vi "UHR-Fleezers Control (fpga) - 9.1.vi"() -> ()   [LabVIEW 2009]
doc: "UHR-Fleezers Instrument Control Code (fpga)"
uses:
  <vilib>/Platform/TimedLoop/XDataNode/XDataNode.xnode
  <vilib>/Platform/TimedLoop/XDataNode/loadlvalarms.vi
  <vilib>/Platform/TimedLoop/XDataNode/timing_clust.ctl
  <vilib>/Platform/TimedLoop/XDataNode/nitl_modes.ctl
  <vilib>/Platform/TimedLoop/XDataNode/wakeup.ctl
  <vilib>/eio/EIOMethodNode/EIOMethodNode.xnode
  <vilib>/rvi/eio/nirviEIOMethodImplementation/nirviEIOMethodImplementation.xnode
  <vilib>/rvi/eio/common/nirviEmuTemplateMethod_noerrors.vi
  <vilib>/rvi/eio/common/nirviEmuClasses.ctl
  <vilib>/eio/EIONode/EIONode.xnode
  <vilib>/rvi/eio/nirviEIOImplementation/nirviEIOImplementation.xnode
  <vilib>/rvi/DataTransferAndStorage/Container/XNode/niFpgaContainer.xnode
  <vilib>/rvi/interface/RandomDataEmulation/niFpgaRandomDataHandleErrors.vi
  <vilib>/rvi/interface/RandomDataEmulation/nirviRandomDataFPGAFIFO.vi
  <vilib>/rvi/DataTransferAndStorage/Container/Common/niFpgaContainerMethod.ctl
  <vilib>/rvi/DataTransferAndStorage/Container/Common/niFpgaTransferTypeControl.ctl
  <vilib>/Platform/TimedLoop/XDataNode/XDNodeRunTimeDep.lvlib
panel:
  in  "Tab Control":T1(tab)=enum."Green Laser Interlacing"
  in  "AI Averages":u16=1 min=1 step=1
  in  "AI1 Sets to FIFO":T2={"Set 1"=TRUE, "Set 2"=TRUE, "Set 3"=FALSE}
  in  "N of AI1 Int Acq Sets":i16=2 min=1 max=3 step=1
  out "Number of AI channels":i16
  out "AI Late Counter":u32
  in  "ai count":u32=400
  out "AI late?":bool
  in  "+ phase":bool
  in  "Phase count adjustment":i16
  out "Relative phase":i16
  in  "DMA buffer timeout":i32
  in  "AI to FIFO":bool
  in  "Tab Control 2":T3(tab)
  in  "Swap F1 and F2":bool
  in  "Freq or Amp switch first":bool=TRUE
  in  "Cont. Scan":bool
  in  "Abort scan":bool
  in  "Cycles per step":u64
  in  "Scan BD":bool
  in  "Number of scans":u16
  in  "Scan steps":u64
  in  "Scan freq.  increment":i64
  out "Scanning":bool
  in  "Start scan":bool
  in  "OSK Bd 1":bool
  in  "Reset Bd 1":bool
  in  "RD":bool
  in  "PMODE":bool
  in  "OSK Bd 2":bool
  in  "Reset Bd 2":bool
  in  "Direct RF Box \nCommunication":bool
  in  "Data BD 2":u8 format="%08b"
  in  "Data BD 1":u8 format="%08b"
  in  "Address":u8 format="%02x"
  in  "Update Data":bool
  in  "FPGA Controls\n RF Box":bool
  in  "Number Interlace Cycles":u8=2 min=1 max=3
  in  "Interlace Off Parameters":u8=1 min=1 max=3
  in  "Interlace ON/OFF":bool
  out "DIO Relative phase":i16
  in  "Phase count adjustment (DIO)":i16
  in  "+ phase (DIO)":bool
  out "DIO Late Counter":u32
  out "DIO Late?":bool
  in  "DIO count 1 (ticks)":u32=400
  in  "DIO count 2 (ticks)":u32=400
  in  "DIO count 3 (ticks)":u32=400
  out "AI2 Y Sum Set 2":i16
  out "AI2 Y Sum Set 1":i16
  in  "FB Gains Set 1":T4={"proportional gain (Kc)"=10, "integral gain (Kc*Ts/Ti)"=5, "derivative gain (Kc*Td/Ts)"=0}
  in  "FB Setpoint Set 1":i16 min=0 step=1
  in  "FB Reset Set 1":bool
  in  "FB On/Off Set 1":bool
  in  "FB Reset Set 2":bool
  in  "FB On/Off Set 2":bool
  in  "FB Setpoint Set 2":i16 min=0 step=1
  in  "FB Gains Set 2":T4={"proportional gain (Kc)"=10, "integral gain (Kc*Ts/Ti)"=5, "derivative gain (Kc*Td/Ts)"=0}
  in  "FB output range 2":cluster{"output high":i16, "output low":i16}={"output high"=3000, "output low"=0}
  in  "FB output range 1":cluster{"output high":i16, "output low":i16}={"output high"=3000, "output low"=0}
  out "Scan I":u64
  in  "Amp switch delay":u16=5
  in  "Freq switch delay":u16
  in  "BD 2 Amplitude 1":u16
  in  "BD 1 Amplitude 1":u16
  in  "BD 2 Frequency 1":u64
  in  "BD 1 Frequency 1":u64
  in  "BD 2 Amplitude 2":u16
  in  "BD 1 Amplitude 2":u16
  in  "BD 2 Frequency 2":u64
  in  "BD 1 Frequency 2":u64
  in  "BD 2 Amplitude 3":u16
  in  "BD 1 Amplitude 3":u16
  in  "BD 2 Frequency 3":u64
  in  "BD 1 Frequency 3":u64
  out "Numeric":i32
  out "AO2 2":i16
  out "AO1 2":i16
  in  "1D or 2D Scan?":bool
  in  "Abort scan (MCL)":bool
  in  "MCL Scan Axis":bool
  in  "Cont. Scan (MCL)":bool
  out "Scan I (MCL)":u64
  in  "Number of scans (MCL)":u16
  out "Scanning MCL":bool
  in  "Scan steps (MCL)":u64
  in  "Cycles per step (MCL)":u64
  in  "Scan freq.  increment (MCL)":i16
  in  "Start scan (MCL)":bool
  in  "AO2":i16
  in  "AO1":i16
  out "MCL Late Counter":u32
  out "MCL Late?":bool
  in  "MCL count":u32=800
  out "MCL Relative Phase":i16
  in  "Phase count adjustment (MCL)":i16
  in  "+ phase (MCL)":bool
  in  "APD Gate Operating Mode":u8 max=2 step=1
  in  "Invert APD Gate":bool
  in  "APD Gate OFF Count":u32=100
  in  "APD Gate ON Count":u32=300
  out "APD Gate Late Counter":u32
  out "APD Gate Late?":bool
  out "APD Gate Relative Phase":i16
  in  "Phase count adjustment (APD Gate)":i16
  in  "+ phase (APD Gate)":bool
  out "APD 2 Counts 0":u32
  out "APD 2 Counts 1":u32
  out "APD 1 Counts 0":u32
  out "APD 1 Counts 1":u32
  out "APD out state":bool
  in  "APD 2 AO offset":i16
  in  "APD 1 AO offset":i16
  in  "APD 2 AO scale factor":i16=1
  in  "APD 1 AO scale factor":i16=1
  in  "APD to FIFO":bool
  in  "APD Acq Rate Count":u32=20000000
  out "APD Acq Late Counter":u32
  out "APD Acq Late?":bool
  out "APD Acq Relative Phase":i16
  in  "Phase Count Adjustment (APD Acq)":i16
  in  "+ phase (APD Acq)":bool
  out "Green FB Signals":T5
  in  "Green FB Count":u32=1200
  out "Green Late Counter":u32
  out "Green FB Late?":bool
  out "Green FB Relative Phase":i16
  in  "Phase count adjustment (Green FB)":i16=10
  in  "+ phase (Green FB)":bool
  out "Green FB Sum":i16
  in  "Green int current ON count adj":u32=150
  in  "Current Out":u16=30000
  in  "Green FB On/Off":bool
  in  "Green FB Setpoint":i16=250 min=0 step=1
  in  "Green FB Gains":T4={"proportional gain (Kc)"=10, "integral gain (Kc*Ts/Ti)"=5, "derivative gain (Kc*Td/Ts)"=0}
  in  "Green FB Reset":bool
  in  "Operating Mode 2":u8=2 max=2 step=1
  in  "Invert GI 2":bool
  in  "Green interlace OFF count 2":u32=900
  in  "Green interlace ON count 2":u32=300
  out "GI Late Counter 2":u32
  out "GI Late? 2":bool
  out "GI Relative phase 2":i16
  in  "Phase count adjustment (GI) 2":i16=20
  in  "+ phase (GI) 2":bool
  in  "Green interlace OFF count":u32=100
  out "GI Relative phase":i16
  in  "Phase count adjustment (GI)":i16
  in  "+ phase (GI)":bool
  out "GI Late?":bool
  in  "Green interlace ON count":u32=300
  out "GI Late Counter":u32
  in  "Invert GI":bool
  in  "Operating Mode":u8 max=2 step=1
  # "Only one of these can be on\nat a time:"
  # "Raster Scan AOD"
  # "1 (X)"
  # "2 (Y)"
  # "IR Intensity Feedback (RF BD 1)"
  # "AO1 (Y)"
  # "2D"
  # "1D"
  # "AO2 (X)"
  # "APD AO for aligning"
  # "Detection Loop"
  # "Green fluorescent laser digital gate interlacing loop"
  # "0 Forced ON\n1 Forced OFF\n2 Interlacing"
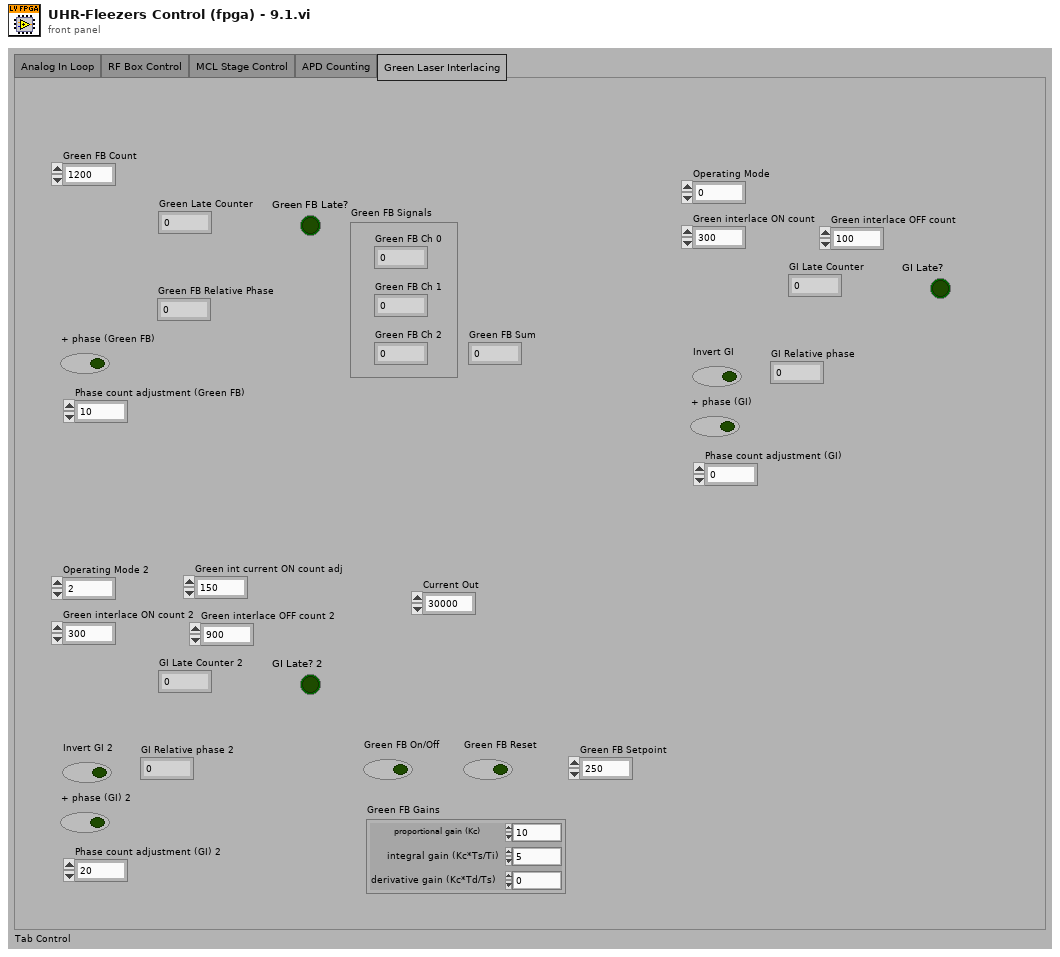
[diagram p1: front panel]
types:
  T1 = enum32{"Analog In Loop", "RF Box Control", "MCL Stage Control", "APD Counting", "Green Laser Interlacing"}
  T2 = cluster{"Set 1":bool, "Set 2":bool, "Set 3":bool}
  T3 = enum32{"Controls", "Interlacing Frequency and Amplitude Values"}
  T4 = cluster{"proportional gain (Kc)":i16, "integral gain (Kc*Ts/Ti)":i16, "derivative gain (Kc*Td/Ts)":i16}
  T5 = cluster{"Green FB Ch 0":i16, "Green FB Ch 1":i16, "Green FB Ch 2":i16}
  T6 = typedef "nirviEmuClasses.ctl" = enum16{"IO Read", "IO Write", "Method", "Property Read", "Property Write"}
  T7 = typedef "XDNodeRunTimeDep.lvlib/timing_clust.ctl" = cluster{"Expected End [f-1]":u64, "Actual End [f-1]":u64, "Finished Late? [f-1]":bool, "Expected End [i-1]":u64, "Actual End [i-1]":u64, "Finished Late? [i-1]":bool, "Expected Start [i]":u64, "Actual Start [i]":u64, "Expected Start [f]":u64, "Actual Start [f]":u64, "Source Name":string, "Structure Name":string, "Period":i64, "Deadline":i64, "Offset":i64, "Start":i64, "Priority":i32, "Timeout":i32, "Mode":T8, "Wakeup Reason":T9, "Error":errorcluster, "Source Type":string, "Secondary Source Type":string, "Global End Time":u64, "Global Start Time":u64, "Frame Duration":u64, "Iteration Duration":u64, "Assigned CPU":i32, "I/O Scan Engine Mode":u32}
  T8 = typedef "XDNodeRunTimeDep.lvlib/nitl_modes.ctl" = enum32{"No Change", "Process missed periods, maintain original phase", "Discard missed periods, maintain original phase", "Process missed periods, ignore original phase", "Discard missed periods, ignore original phase"}
  T9 = typedef "XDNodeRunTimeDep.lvlib/wakeup.ctl" = enum32{"Normal", "Aborted", "Asynchronous wakeup", "Timing source error", "Timed loop error", "Timeout"}
  T10 = typedef "niFpgaContainerMethod.ctl" = enum16{"Write", "Read", "Clear", "Get Number of Elements to Write", "Get Number of Elements to Read", "Enable", "Disable", "Flush and Disable", "Get Stream State"}
  T11 = typedef "niFpgaTransferTypeControl.ctl" = enum16{"Target-Scoped", "Host to Target - DMA", "Target to Host - DMA", "Peer to Peer Reader", "Peer to Peer Writer", "Bidirectional"}
  T12 = cluster{"Chassis2/Mod1/AI0":i16, "Chassis2/Mod1/AI1":i16, "Chassis2/Mod1/AI2":i16}
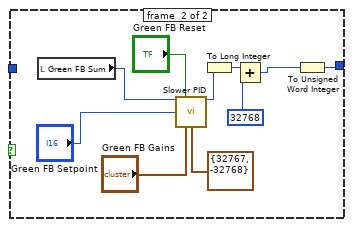
[diagram p2: hidden frame]
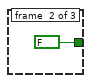
[diagram p3: hidden frame]
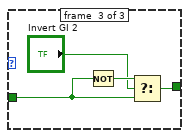
[diagram p4: hidden frame]
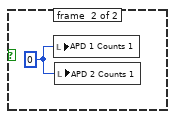
[diagram p5: hidden frame]
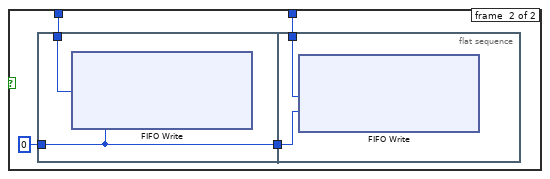
[diagram p6: hidden frame]
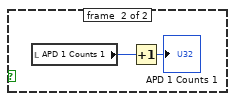
[diagram p7: hidden frame]
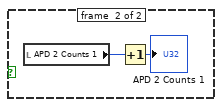
[diagram p8: hidden frame]
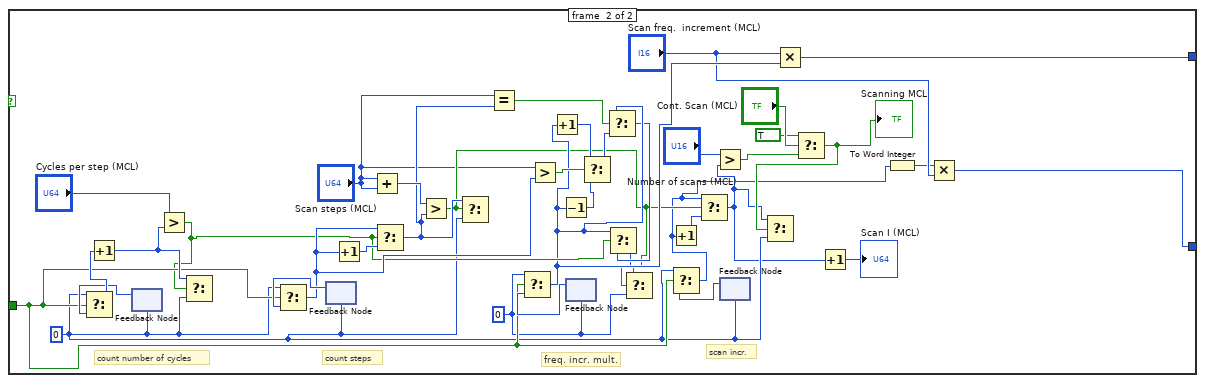
[diagram p9: hidden frame]
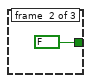
[diagram p10: hidden frame]
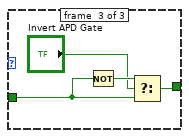
[diagram p11: hidden frame]
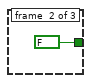
[diagram p12: hidden frame]
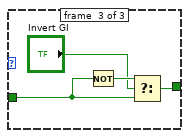
[diagram p13: hidden frame]
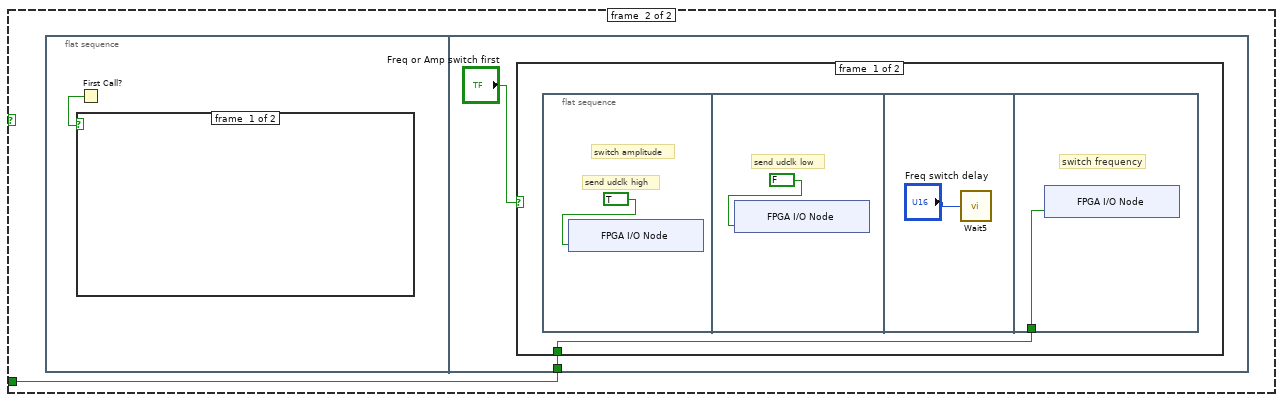
[diagram p14: hidden frame]
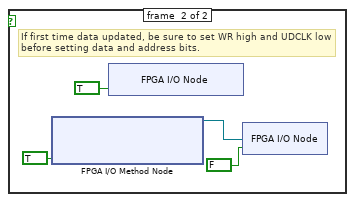
[diagram p15: hidden frame]
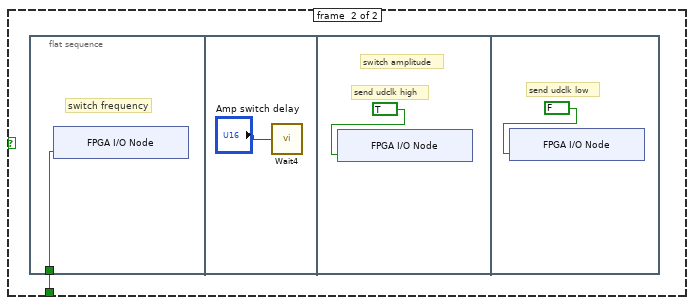
[diagram p16: hidden frame]
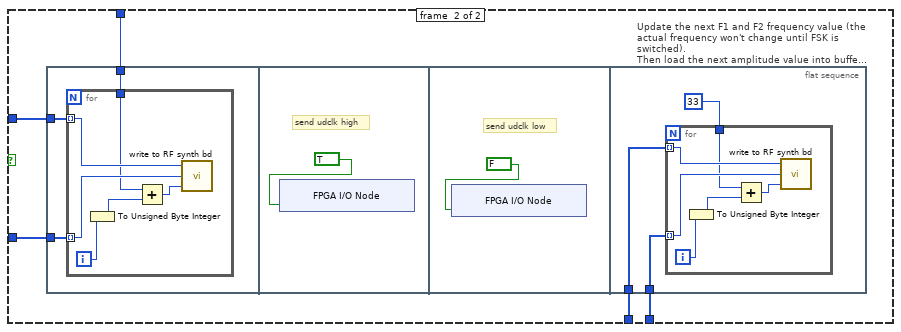
[diagram p17: hidden frame]
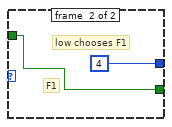
[diagram p18: hidden frame]
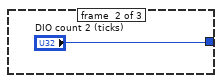
[diagram p19: hidden frame]
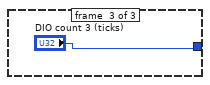
[diagram p20: hidden frame]
diagram:
  # "timing array current index"
  # "timing array"
  # "timing counter (phase adjusted here)"
  # "late counter"
  n1 = flat-sequence "FPGA initialization to do before running any of the loops" {
    tunnel: [u32 0 ("DIO count 3 (ticks)")] -> w1
    tunnel: [w10] -> _
    frame #0 {
      # "This is a kludge to let host programs know how many channels of data are in the DMA stream.  Set by hand."
      # "Start up expansion chassis early\nto avoid delays later"
      # "This pin controls udclk on the RF boards.\nWhen initially configuring the boards, this pin needs to be\nconfigured as a high impedance input.  Later it will be switched\nto an output."
      # "Initial setting of DIO data and \naddress to low (before reset).  \nThis needs to happen before the other\ncontrol method loops execute."
      n2 = xnode "FPGA I/O Node"("Chassis2/Mod4/AO0"=u16 0) -> ("Chassis2/Mod1/AI0"=w10:i16)  [unwired: 2 in, 2 out]
      n3 = xnode "FPGA I/O Method Node"("Enable"=FALSE) -> ()  [unwired: 1 in, 1 out]
      n4 = xnode "FPGA I/O Node"("Connector1/DIO0"=FALSE, "Connector1/DIO1"=FALSE, "Connector1/DIO2"=FALSE, "Connector1/DIO3"=FALSE, "Connector1/DIO4"=FALSE, "Connector1/DIO5"=FALSE, "Connector1/DIO6"=FALSE, "Connector1/DIO7"=FALSE, "Connector1/DIO8"=FALSE, "Connector1/DIO9"=FALSE, "Connector1/DIO10"=FALSE, "Connector1/DIO11"=FALSE, "Connector1/DIO12"=FALSE, "Connector1/DIO13"=FALSE, "Connector1/DIO15"=FALSE, "Connector1/DIO20"=FALSE, "Connector1/DIO21"=FALSE, "Connector1/DIO22"=FALSE, "Connector1/DIO23"=FALSE, "Connector1/DIO24"=FALSE, "Connector1/DIO25"=FALSE, "Connector1/DIO26"=FALSE, "Connector1/DIO27"=FALSE, "Connector1/DIO14"=FALSE) -> ()  [unwired: 24 in, 24 out]
      "Number of AI channels" <- i16 12 ("Number of AI channels")
    }
  }
  n5 = node-c288() -> (w3:T7)  [unwired: 1 in]
  n6 = local read "AO1"() -> (w5:i16)
  n7 = local read "AO2"() -> (w4:i16)
  n8 = timed-loop "RF box board DIO control: control bits" {
    timing: w3 -> [_]
    timing-out: [_] -> w2
    tunnel: [w393] -> _
    tunnel: w1 -> [w393]
    stop <- FALSE stop-if-true
    n9 = xnode "FPGA I/O Node"("Connector1/DIO16"="RD", "Connector1/DIO17"="PMODE", "Connector1/DIO18"="OSK Bd 1", "Connector1/DIO19"="Reset Bd 1", "Connector1/DIO28"="OSK Bd 2", "Connector1/DIO29"="Reset Bd 2") -> ()  [unwired: 6 in, 6 out]
  }
  n10 = while "DAQ AI set 1" {
    shift-right: [w481] -> _
    shift-left: w1 -> [w486]
    stop <- FALSE stop-if-true
    n11 = flat-sequence {
      tunnel: w486 -> [w496]
      tunnel: [w497] -> w484
      tunnel: [w496] -> w483
      tunnel: [w507] -> w494
      tunnel: [w506] -> w493
      tunnel: [w505] -> w492
      tunnel: [w504] -> w491
      tunnel: [w503] -> w490
      tunnel: [w502] -> w489
      tunnel: [w501] -> w488
      tunnel: [w500] -> w487
      tunnel: [w499] -> w485
      tunnel: w484 -> [w499]
      tunnel: w483 -> [w498]
      tunnel: [w498] -> w482
      tunnel: [w684] -> w481
      tunnel: w494 -> [w722]
      tunnel: w493 -> [w721]
      tunnel: w492 -> [w705]
      tunnel: w491 -> [w720]
      tunnel: w490 -> [w709]
      tunnel: w489 -> [w708]
      tunnel: w488 -> [w707]
      tunnel: w487 -> [w706]
      tunnel: w485 -> [w701]
      tunnel: w482 -> [w698]
      frame #0 {
        n12 = call "Loop Timer3"("Count(Ticks)"=w496) -> ("Tick Count(Ticks)"=w497:u32)
      }
      frame #1 {
        n13 = xnode "FPGA I/O Node"("Connector1/DIO31"=TRUE ("Connector1/DIO33")) -> ("Connector0/AI0"=w507:i16, "Connector0/AI1"=w506:i16, "Connector0/AI2"=w505:i16, "Connector0/AI3"=w504:i16, "Connector0/AI4"=w503:i16, "Connector0/AI5"=w502:i16, "Connector0/AI6"=w501:i16, "Connector0/AI7"=w500:i16)  [unwired: 9 in, 9 out]
      }
      frame #2 {
        # "Adjust phase after data acquired if button pressed"
        n14 = feedback #1(i16 1) -> (w713:i16)
        n15 = Increment(x=w713) -> (x+1=w719:i16)
        n16 = Greater?(x=w719, y="N of AI1 Int Acq Sets") -> (0:w716:bool)
        n17 = Select(t=i16 1, s=w716, f=w719) -> (s? t:f=w718:i16)
        n18 = feedback #2(FALSE ("AI to FIFO")) -> (w703:bool)
        n19 = case shown="1, Default" w713 {
          tunnel: w705 -> [w725 w729 _]
          tunnel: "AI1 Sets to FIFO" -> [w727 w731 w734]
          tunnel: [w726 w730 w733] -> w710
          tunnel: ["AI to FIFO" w728 w732] -> w702
          tunnel: w703 -> [_ w728 w732]
          frame #0 {
            n20 = Unbundle By Name(w727) -> ("Set 1"=w726:bool)
            "AI2 Y Sum Set 1" <- w725
          }
          frame #1 {
            n21 = Unbundle By Name(w731) -> ("Set 2"=w730:bool)
            "AI2 Y Sum Set 2" <- w729
          }
          frame #2 {
            n22 = Unbundle By Name(w734) -> ("Set 3"=w733:bool)
          }
        }
        n23 = And(x=w710, y=w702) -> (x .and. y?=w712:bool)
        n24 = case shown="True" w712 {
          tunnel: w722 -> [_ w739]
          tunnel: w721 -> [_ w740]
          tunnel: w705 -> [_ w741]
          tunnel: w720 -> [_ w742]
          tunnel: w709 -> [_ w746]
          tunnel: w708 -> [_ w745]
          tunnel: w707 -> [_ w744]
          tunnel: w706 -> [_ w743]
          frame #0 {
          }
          frame #1 {
            n25 = Greater?(x="AI Averages", y=u16 1) -> (0:w737:bool)
            n26 = case shown="True" w737 {
              tunnel: w746 -> [w757 w814]
              tunnel: w745 -> [w756 w813]
              tunnel: w744 -> [w755 w812]
              tunnel: w743 -> [w754 w811]
              tunnel: w742 -> [w753 w810]
              tunnel: w741 -> [w758 w809]
              tunnel: w740 -> [w759 w808]
              tunnel: w739 -> [w760 w807]
              tunnel: "AI Averages" -> [_ w794]
              tunnel: "DMA buffer timeout" -> [w748 w791]
              frame #0 {
                n27 = Join Numbers(hi=w760, lo=w759) -> ((hi.lo)=w752:u32)
                n28 = Join Numbers(hi=w758, lo=w753) -> ((hi.lo)=w751:u32)
                n29 = Join Numbers(hi=w757, lo=w756) -> ((hi.lo)=w750:u32)
                n30 = Join Numbers(hi=w755, lo=w754) -> ((hi.lo)=w749:u32)
                n31 = Build Array(w752, w751, w750, w749) -> (w747:u32[])
                n32 = for {
                  tunnel: w747 -> [w762] mode=indexing
                  tunnel: w748 -> [w763]
                  n33 = To Unsigned Long Integer(number=w762) -> (unsigned 32bit integer=w761:u32)
                  n34 = xnode ("FIFO Write")("Element"=w761, "Timeout"=w763) -> ()  [unwired: 1 in, 2 out]
                }
              }
              frame #1 {
                w798 = u16 0
                n35 = To Long Integer(number=w807) -> (32bit integer=w800:i32)
                n36 = To Long Integer(number=w808) -> (32bit integer=w817:i32)
                n37 = To Long Integer(number=w809) -> (32bit integer=w816:i32)
                n38 = To Long Integer(number=w810) -> (32bit integer=w815:i32)
                n39 = To Long Integer(number=w814) -> (32bit integer=w806:i32)
                n40 = To Long Integer(number=w813) -> (32bit integer=w805:i32)
                n41 = To Long Integer(number=w812) -> (32bit integer=w804:i32)
                n42 = To Long Integer(number=w811) -> (32bit integer=w803:i32)
                n43 = Build Array(w800, w817, w816, w815, w806, w805, w804, w803) -> (w789:i32[])
                n44 = feedback #3(w789) -> (w802:i32[])
                n45 = Add(x=w789, y=w802) -> (x+y=w801:i32[])
                n46 = feedback #4(w798) -> (w796:u16)
                n47 = Increment(x=w796) -> (x+1=w793:u16)
                n48 = Equal?(x=w793, y=u16 1) -> (x = y?=w792:bool)
                n49 = Select(t=w789, s=w792, f=w801) -> (s? t:f=w790:i32[])
                n50 = Greater Or Equal?(x=w793, y=w794) -> (x >= y?=w795:bool)
                n51 = Select(t=w798, s=w795, f=w793) -> (s? t:f=w797:u16)
                n52 = case shown="True" w795 {
                  tunnel: w790 -> [_ w819]
                  tunnel: w791 -> [_ w818]
                  frame #0 {
                  }
                  frame #1 {
                    n53 = for {
                      tunnel: w819 -> [w821] mode=indexing
                      tunnel: w818 -> [w822]
                      n54 = To Unsigned Long Integer(number=w821) -> (unsigned 32bit integer=w820:u32)
                      n55 = xnode ("FIFO Write")("Element"=w820, "Timeout"=w822) -> ()  [unwired: 1 in, 2 out]
                    }
                  }
                }
              }
            }
          }
        }
        n56 = feedback #5(w701) -> (w700:u32)
        n57 = Subtract(x=w701, y=w700) -> (x-y=w699:u32)
        n58 = Subtract(x=w699, y=w698) -> (x-y=w695:u32)
        n59 = Subtract(x="ai count", y=w695) -> (x-y=w685:u32)
        n60 = Greater?(x=w695, y=u32 0) -> (0:w693:bool)
        "AI late?" <- w693
        n61 = feedback #6(u32 0) -> (w691:u32)
        n62 = Increment(x=w691) -> (x+1=w690:u32)
        n63 = Select(t=w690, s=w693, f=w691) -> (s? t:f=w692:u32)
        "AI Late Counter" <- w692
        n64 = xnode "I/O Node"("Connector1/DIO31"=FALSE ("Connector1/DIO34")) -> ()  [unwired: 1 in, 1 out]
        n65 = Boolean To (0,1)(Boolean="+ phase") -> (0, 1=w687:i16)
        n66 = Multiply(x=w687, y="Phase count adjustment") -> (x*y=w681:i16)
        n67 = feedback #7(i16 0) -> (w683:i16)
        n68 = Add(x=w685, y=w681) -> (x+y=w684:u32)
        n69 = Subtract(x=w683, y=w681) -> (x-y=w682:i16)
        "Relative phase" <- w682
      }
    }
  }
  n70 = while "APD 1 Counter" {
    tunnel: w1 -> [_]
    stop <- FALSE stop-if-true
    n71 = flat-sequence {
      frame #0 {
        n72 = xnode "FPGA I/O Method Node"("FPGA I/O In"=refnum<k21> "Connector0/DIO10" ("APD 1 DO"), "Timeout"=-1) -> ()  [unwired: 2 out]
      }
      frame #1 {
        n73 = local read "APD out state"() -> (w887:bool)
        n74 = case shown="False" w887 {
          frame #0 {
            n75 = local read "APD 1 Counts 0"() -> (w889:u32)
            n76 = Increment(x=w889) -> (x+1=→"APD 1 Counts 0":u32)
          }
          frame #1 {
            n77 = local read "APD 1 Counts 1"() -> (w891:u32)
            n78 = Increment(x=w891) -> (x+1=→"APD 1 Counts 1":u32)
          }
        }
      }
    }
  }
  n79 = while "APD 2 Counter" {
    tunnel: w1 -> [_]
    stop <- FALSE stop-if-true
    n80 = flat-sequence {
      frame #0 {
        n81 = xnode "FPGA I/O Method Node"("FPGA I/O In"=refnum<k21> "Connector0/DIO11" ("APD 2 DO"), "Timeout"=-1) -> ()  [unwired: 2 out]
      }
      frame #1 {
        n82 = local read "APD out state"() -> (w918:bool)
        n83 = case shown="False" w918 {
          frame #0 {
            n84 = local read "APD 2 Counts 0"() -> (w920:u32)
            n85 = Increment(x=w920) -> (x+1=→"APD 2 Counts 0":u32)
          }
          frame #1 {
            n86 = local read "APD 2 Counts 1"() -> (w922:u32)
            n87 = Increment(x=w922) -> (x+1=→"APD 2 Counts 1":u32)
          }
        }
      }
    }
  }
  n88 = while "RF box board DIO control: parallel communication" {
    shift-right: [w929] -> _
    shift-left: w1 -> [w928]
    shift-right: [w927] -> _
    shift-left: FALSE ("Swap F1 and F2") -> [w926]
    stop <- FALSE stop-if-true
    n89 = flat-sequence {
      tunnel: w926 -> [w933]
      tunnel: w928 -> [w931]
      tunnel: [w933] -> w925
      tunnel: [w932] -> w924
      tunnel: [w931] -> w923
      tunnel: [w939] -> w929
      tunnel: [w938] -> w927
      tunnel: w925 -> [w937]
      tunnel: w924 -> [w935]
      tunnel: w923 -> [w934]
      frame #0 {
        n90 = call "Loop Timer"("Count(Ticks)"=w931) -> ("Tick Count(Ticks)"=w932:u32)
      }
      frame #1 {
        n91 = flat-sequence {
          tunnel: ["FPGA Controls\n RF Box"] -> w936
          tunnel: w937 -> [w940]
          tunnel: [w1089] -> w939
          tunnel: [w1109] -> w938
          tunnel: w936 -> [w1108]
          tunnel: w935 -> [w1102]
          tunnel: w934 -> [w1099]
          frame #0 {
            n92 = case shown="True" "FPGA Controls\n RF Box" {
              tunnel: w940 -> [_ w942]
              frame #0 {
              }
              frame #1 {
                n93 = flat-sequence {
                  tunnel: w942 -> [w987]
                  frame #0 {
                    n94 = First Call?() -> (First Call?: T/F=w943:bool)
                    n95 = case shown="True" w943 {
                      frame #0 {
                      }
                      frame #1 {
                        # "If first time data updated, be sure to set WR high and UDCLK low\nbefore setting data and address bits."
                        n96 = xnode "FPGA I/O Method Node"("Enable"=TRUE) -> ("FPGA I/O Out"=w945:refnum<k21>)  [unwired: 1 in]
                        n97 = xnode "FPGA I/O Node"("Connector1/DIO15"=TRUE) -> ()  [unwired: 1 in, 1 out]
                        n98 = xnode "FPGA I/O Node"("I/O Item"=FALSE ("Connector1/DIO30"), "FPGA I/O In"=w945) -> ()  [unwired: 1 out]
                      }
                    }
                  }
                  frame #1 {
                    n99 = case shown="True" "Freq or Amp switch first" {
                      tunnel: w987 -> [w989 w1033]
                      frame #0 {
                        n100 = flat-sequence {
                          tunnel: w989 -> [w1019]
                          frame #0 {
                            # "switch amplitude"
                            # "send udclk high"
                            n101 = xnode "FPGA I/O Node"("Connector1/DIO30"=TRUE ("Connector1/DIO15")) -> ()  [unwired: 1 in, 1 out]
                          }
                          frame #1 {
                            # "send udclk low"
                            n102 = xnode "FPGA I/O Node"("Connector1/DIO30"=FALSE ("Connector1/DIO15")) -> ()  [unwired: 1 in, 1 out]
                          }
                          frame #2 {
                            n103 = call "Wait5"("Count(Ticks)"="Freq switch delay") -> ()  [unwired: 1 out]
                          }
                          frame #3 {
                            # "switch frequency"
                            n104 = xnode "FPGA I/O Node"("Connector1/DIO36"=w1019) -> ()  [unwired: 1 in, 1 out]
                          }
                        }
                      }
                      frame #1 {
                        n105 = flat-sequence {
                          tunnel: w1033 -> [w1034]
                          frame #0 {
                            # "switch frequency"
                            n106 = xnode "FPGA I/O Node"("Connector1/DIO36"=w1034) -> ()  [unwired: 1 in, 1 out]
                          }
                          frame #1 {
                            n107 = call "Wait4"("Count(Ticks)"="Amp switch delay") -> ()  [unwired: 1 out]
                          }
                          frame #2 {
                            # "switch amplitude"
                            # "send udclk high"
                            n108 = xnode "FPGA I/O Node"("Connector1/DIO30"=TRUE ("Connector1/DIO15")) -> ()  [unwired: 1 in, 1 out]
                          }
                          frame #3 {
                            # "send udclk low"
                            n109 = xnode "FPGA I/O Node"("Connector1/DIO30"=FALSE ("Connector1/DIO15")) -> ()  [unwired: 1 in, 1 out]
                          }
                        }
                      }
                    }
                  }
                }
              }
            }
          }
          frame #1 {
            # "This is the prior cycle's on time"
            # "increment timing\nindex, reset to 0 if \nend of matrix"
            # "Reset to begginning (1) when number of cycles reached."
            # "timing index"
            # "build byte stacks for writing data\n(must correspond to addresses array constant)"
            # "Timing housekeeping"
            # "Adjust phase if late\n(maintains constant phase relationship between cycles)"
            n110 = feedback #8(u8 0 ("t")) -> (w1105:u8)
            n111 = Increment(x=w1105) -> (x+1=w1149:u8)
            n112 = Increment(x="Number Interlace Cycles") -> (x+1=w1144:u8)
            n113 = Equal?(x=w1149, y=w1144) -> (x = y?=w1151:bool)
            n114 = Select(t=u8 1, s=w1151, f=w1149) -> (s? t:f=w1104:u8)
            n115 = Increment(x=w1104) -> (x+1=w1146:u8)
            n116 = Equal?(x=w1146, y=w1144) -> (x = y?=w1147:bool)
            n117 = Select(t=u8 1, s=w1147, f=w1146) -> (s? t:f=w1143:u8)
            n118 = Select(t=w1143, s="Interlace ON/OFF", f="Interlace Off Parameters") -> (s? t:f=w1127:u8)
            n119 = case shown="1, Default" w1127 {
              tunnel: [w1223 "BD 1 Frequency 2" "BD 1 Frequency 3"] -> w1139
              tunnel: [w1222 "BD 2 Frequency 2" "BD 2 Frequency 3"] -> w1128
              tunnel: ["BD 2 Amplitude 1" "BD 2 Amplitude 2" "BD 2 Amplitude 3"] -> w1077
              tunnel: [w1211 w1281 "BD 1 Amplitude 3"] -> w1080
              frame #0 {
                w1218 = u8 0 ("f")
                n120 = local read "Scanning"() -> (w1224:bool)
                n121 = Or(x=w1224, y="Start scan") -> (x .or. y?=w1216:bool)
                n122 = Not(x="Abort scan") -> (.not. x?=w1214:bool)
                n123 = And(x=w1214, y=w1216) -> (x .and. y?=w1213:bool)
                n124 = case "Raster scan" shown="True" w1213 {
                  tunnel: [i16 0 w1270] -> w1219
                  tunnel: "Start scan" -> [_ w1255]
                  frame #0 {
                    n125 = local write "Scanning"(FALSE ("scanning")) -> ()
                  }
                  frame #1 {
                    w1239 = i64 0
                    w1238 = u64 0
                    # "scan incr."
                    # "freq. incr. mult."
                    # "count steps"
                    # "count number of cycles"
                    n126 = feedback #9(w1238) -> (w1267:u64)
                    n127 = Select(t=w1238, s=w1255, f=w1267) -> (s? t:f=w1269:u64)
                    n128 = Increment(x=w1269) -> (x+1=w1266:u64)
                    n129 = Greater?(x="Cycles per step", y=w1266) -> (0:w1248:bool)
                    n130 = Select(t=w1266, s=w1248, f=w1238) -> (s? t:f=w1265:u64)
                    n131 = feedback #10(w1238) -> (w1264:u64)
                    n132 = Select(t=w1238, s=w1255, f=w1264) -> (s? t:f=w1259:u64)
                    n133 = Increment(x=w1259) -> (x+1=w1263:u64)
                    n134 = Add(x="Scan steps", y="Scan steps") -> (x+y=w1262:u64)
                    n135 = Select(t=w1259, s=w1248, f=w1263) -> (s? t:f=w1243:u64)
                    n136 = Greater?(x=w1262, y=w1243) -> (0:w1242:bool)
                    n137 = Select(t=w1243, s=w1242, f=w1238) -> (s? t:f=w1260:u64)
                    n138 = Equal?(x="Scan steps", y=w1243) -> (x = y?=w1247:bool)
                    n139 = Greater?(x="Scan steps", y=w1259) -> (0:w1258:bool)
                    n140 = feedback #11(w1239) -> (w1261:i64)
                    n141 = Select(t=w1239, s=w1255, f=w1261) -> (s? t:f=w1245:i64)
                    n142 = Increment(x=w1245) -> (x+1=w1257:i64)
                    n143 = Decrement(x=w1245) -> (x-1=w1256:i64)
                    n144 = Select(t=w1257, s=w1258, f=w1256) -> (s? t:f=w1246:i64)
                    n145 = Select(t=w1245, s=w1247, f=w1246) -> (s? t:f=w1244:i64)
                    n146 = Select(t=w1245, s=w1248, f=w1244) -> (s? t:f=w1240:i64)
                    n147 = Select(t=w1240, s=w1242, f=w1239) -> (s? t:f=w1241:i64)
                    n148 = feedback #12(w1238) -> (w1254:u64)
                    n149 = Select(t=w1238, s=w1255, f=w1254) -> (s? t:f=w1250:u64)
                    n150 = Increment(x=w1250) -> (x+1=w1251:u64)
                    n151 = Select(t=w1250, s=w1242, f=w1251) -> (s? t:f=w1249:u64)
                    n152 = Greater?(x="Number of scans", y=w1249) -> (0:w1235:bool)
                    n153 = Multiply(x="Scan freq.  increment", y=w1245) -> (x*y=w1270:i64)
                    n154 = Select(t=TRUE, s="Cont. Scan", f=w1235) -> (s? t:f=w1234:bool)
                    "Scanning" <- w1234
                    n155 = Select(t=w1249, s=w1234, f=w1238) -> (s? t:f=w1252:u64)
                    n156 = Increment(x=w1249) -> (x+1=→"Scan I":u64)
                  }
                }
                n157 = case shown="True" "FB On/Off Set 1" {
                  tunnel: "BD 1 Amplitude 1" -> [w1272 _]
                  tunnel: [w1272 w1273] -> w1211
                  frame #0 {
                  }
                  frame #1 {
                    n158 = local read "AI2 Y Sum Set 1"() -> (w1275:i16)
                    n159 = call "Slower PID.vi"("process variable"=w1275, "reset?"="FB Reset Set 1", "setpoint"="FB Setpoint Set 1", "PID gains (x 2^8)"="FB Gains Set 1", "output range"="FB output range 1") -> ("output"=w1278:i16)  [unwired: 10 out]
                    n160 = To Unsigned Word Integer(number=w1278) -> (unsigned 16bit integer=w1273:u16)
                  }
                }
                n161 = Select(t=w1218, s="Scan BD", f=w1219) -> (s? t:f=w1217:i64)
                n162 = Select(t=w1219, s="Scan BD", f=w1218) -> (s? t:f=w1220:i64)
                n163 = Add(x=w1217, y="BD 2 Frequency 1") -> (x+y=w1222:u64)
                n164 = Add(x="BD 1 Frequency 1", y=w1220) -> (x+y=w1223:u64)
              }
              frame #1 {
                n165 = case shown="True" "FB On/Off Set 2" {
                  tunnel: [w1286 w1287] -> w1281
                  tunnel: "BD 1 Amplitude 2" -> [w1286 _]
                  frame #0 {
                  }
                  frame #1 {
                    n166 = local read "AI2 Y Sum Set 2"() -> (w1292:i16)
                    n167 = call "Slower PID.vi"("process variable"=w1292, "reset?"="FB Reset Set 2", "setpoint"="FB Setpoint Set 2", "PID gains (x 2^8)"="FB Gains Set 2", "output range"="FB output range 2") -> ("output"=w1289:i16)  [unwired: 10 out]
                    n168 = To Unsigned Word Integer(number=w1289) -> (unsigned 16bit integer=w1287:u16)
                  }
                }
              }
              frame #2 {
              }
            }
            n169 = feedback #13(w1102) -> (w1101:u32)
            n170 = Subtract(x=w1102, y=w1101) -> (x-y=w1100:u32)
            n171 = Select(t=w1104, s="Interlace ON/OFF", f="Interlace Off Parameters") -> (s? t:f=w1142:u8)
            n172 = Subtract "The error"(x=w1100, y=w1099) -> (x-y=w1097:u32)
            n173 = case shown="3" w1142 {
              tunnel: ["DIO count 1 (ticks)" "DIO count 2 (ticks)" "DIO count 3 (ticks)"] -> w1098
              frame #0 {
              }
              frame #1 {
              }
              frame #2 {
              }
            }
            n174 = Greater?(x=w1097, y=u32 0) -> (0:w1092:bool)
            "DIO Late?" <- w1092
            n175 = feedback #14(u32 0) -> (w1094:u32)
            n176 = Increment(x=w1094) -> (x+1=w1093:u32)
            n177 = Select(t=w1093, s=w1092, f=w1094) -> (s? t:f=w1095:u32)
            "DIO Late Counter" <- w1095
            n178 = Subtract(x=w1098, y=w1097) -> (x-y=w1090:u32)
            n179 = Boolean To (0,1)(Boolean="+ phase (DIO)") -> (0, 1=w1087:i16)
            n180 = Multiply(x=w1087, y="Phase count adjustment (DIO)") -> (x*y=w1083:i16)
            n181 = feedback #15(i16 0) -> (w1085:i16)
            n182 = Subtract(x=w1085, y=w1083) -> (x-y=w1084:i16)
            "DIO Relative phase" <- w1084
            n183 = Split Number(x=w1128) -> (hi(x)=w1133:u32, lo(x)=w1132:u32)
            n184 = Split Number(x=w1139) -> (hi(x)=w1138:u32, lo(x)=w1137:u32)
            n185 = Split Number(x=w1133) -> (lo(x)=w1131:u16)  [unwired: 1 out]
            n186 = Split Number(x=w1132) -> (hi(x)=w1130:u16, lo(x)=w1129:u16)
            n187 = Split Number(x=w1138) -> (lo(x)=w1136:u16)  [unwired: 1 out]
            n188 = Split Number(x=w1137) -> (hi(x)=w1135:u16, lo(x)=w1134:u16)
            n189 = Split Number(x=w1080) -> (hi(x)=w1082:u8, lo(x)=w1081:u8)
            n190 = Split Number(x=w1131) -> (hi(x)=w1119:u8, lo(x)=w1118:u8)
            n191 = Split Number(x=w1130) -> (hi(x)=w1117:u8, lo(x)=w1116:u8)
            n192 = Split Number(x=w1129) -> (hi(x)=w1115:u8, lo(x)=w1114:u8)
            n193 = Split Number(x=w1077) -> (hi(x)=w1079:u8, lo(x)=w1078:u8)
            n194 = Add(x=w1090, y=w1083) -> (x+y=w1089:u32)
            n195 = Split Number(x=w1136) -> (hi(x)=w1126:u8, lo(x)=w1125:u8)
            n196 = Split Number(x=w1135) -> (hi(x)=w1124:u8, lo(x)=w1123:u8)
            n197 = Split Number(x=w1134) -> (hi(x)=w1122:u8, lo(x)=w1121:u8)
            n198 = Build Array "BD 1 A Stack"(w1082, w1081) -> (w1111:u8[])
            n199 = Build Array "BD 2 nu Stack"(w1119, w1118, w1117, w1116, w1115, w1114) -> (w1113:u8[])
            n200 = Build Array "BD 2 A Stack"(w1079, w1078) -> (w1110:u8[])
            n201 = Build Array "BD 1 nu Stack"(w1126, w1125, w1124, w1123, w1122, w1121) -> (w1120:u8[])
            n202 = case shown="2" w1127 {
              tunnel: [w1203 w1206] -> w1109
              tunnel: [u8 10 u8 4] -> w1112
              tunnel: "Swap F1 and F2" -> [w1204 w1206]
              frame #0 {
                # "F2"
                n203 = Not(x=w1204) -> (.not. x?=w1203:bool)
              }
              frame #1 {
                # "low chooses F1"
                # "F1"
              }
            }
            n204 = case "If FPGA is controlling (toggling) RF synth" shown="True" w1108 {
              tunnel: w1120 -> [_ w1156]
              tunnel: w1113 -> [_ w1155]
              tunnel: w1112 -> [_ w1154]
              tunnel: w1111 -> [_ w1153]
              tunnel: w1110 -> [_ w1152]
              frame #0 {
              }
              frame #1 {
                n205 = flat-sequence "Update the next F1 and F2 frequency value (the actual frequency won't change until FSK is switched).\nThen load the next amplitude value into buffer, but don't update it until the next cycle." {
                  tunnel: w1156 -> [w1159]
                  tunnel: w1155 -> [w1158]
                  tunnel: w1154 -> [w1157]
                  tunnel: w1153 -> [w1196]
                  tunnel: w1152 -> [w1195]
                  frame #0 {
                    n206 = for {
                      tunnel: w1159 -> [w1165] mode=indexing
                      tunnel: w1158 -> [w1164] mode=indexing
                      tunnel: w1157 -> [w1162]
                      i -> [w1163]
                      n207 = To Unsigned Byte Integer(number=w1163) -> (unsigned 8bit integer=w1160:u8)
                      n208 = Add(x=w1162, y=w1160) -> (x+y=w1161:u8)
                      n209 = call "write to RF synth bd.vi"("Address Byte"=w1161, "BD 2 Byte"=w1164, "BD 1 Byte"=w1165) -> ()
                    }
                  }
                  frame #1 {
                    # "send udclk high"
                    n210 = xnode "FPGA I/O Node"("Connector1/DIO30"=TRUE ("Connector1/DIO15")) -> ()  [unwired: 1 in, 1 out]
                  }
                  frame #2 {
                    # "send udclk low"
                    n211 = xnode "FPGA I/O Node"("Connector1/DIO30"=FALSE ("Connector1/DIO15")) -> ()  [unwired: 1 in, 1 out]
                  }
                  frame #3 {
                    n212 = for {
                      tunnel: w1196 -> [w1202] mode=indexing
                      tunnel: w1195 -> [w1201] mode=indexing
                      tunnel: u8 33 -> [w1199]
                      i -> [w1200]
                      n213 = To Unsigned Byte Integer(number=w1200) -> (unsigned 8bit integer=w1197:u8)
                      n214 = Add(x=w1199, y=w1197) -> (x+y=w1198:u8)
                      n215 = call "write to RF synth bd.vi"("Address Byte"=w1198, "BD 2 Byte"=w1201, "BD 1 Byte"=w1202) -> ()
                    }
                  }
                }
              }
            }
          }
        }
      }
    }
  }
  n216 = while "Control APD data integration - stream to host" {
    shift-right: [w1300] -> _
    shift-left: w1 -> [w1305]
    stop <- FALSE stop-if-true
    n217 = flat-sequence {
      tunnel: w1305 -> [w1307]
      tunnel: [w1308] -> w1303
      tunnel: [w1307] -> w1301
      tunnel: [w1316] -> w1304
      tunnel: w1303 -> [w1316]
      tunnel: [w1315] -> w1302
      tunnel: w1301 -> [w1315]
      tunnel: [w1314] -> w1299
      tunnel: [w1313] -> w1298
      tunnel: [w1340] -> w1300
      tunnel: w1304 -> [w1365]
      tunnel: w1302 -> [w1362]
      tunnel: w1299 -> [w1333]
      tunnel: w1298 -> [w1332]
      frame #0 {
        n218 = call "Loop Timer6"("Count(Ticks)"=w1307) -> ("Tick Count(Ticks)"=w1308:u32)
      }
      frame #1 {
        n219 = flat-sequence {
          tunnel: [w1317] -> w1312
          tunnel: w1312 -> [w1320]
          tunnel: [w1322] -> w1311
          tunnel: [w1321] -> w1310
          tunnel: [w1320] -> w1309
          tunnel: [w1328] -> w1313
          tunnel: [w1329] -> w1314
          tunnel: w1311 -> [w1329]
          tunnel: w1310 -> [w1328]
          tunnel: w1309 -> [w1327]
          frame #0 {
            n220 = feedback #16(FALSE) -> (w1318:bool)
            "APD out state" <- w1318
            n221 = Not(x=w1318) -> (.not. x?=w1317:bool)
          }
          frame #1 {
            n222 = local read "APD 1 Counts 1"() -> (w1326:u32)
            n223 = local read "APD 1 Counts 0"() -> (w1325:u32)
            n224 = local read "APD 2 Counts 1"() -> (w1324:u32)
            n225 = local read "APD 2 Counts 0"() -> (w1323:u32)
            n226 = Select(t=w1326, s=w1320, f=w1325) -> (s? t:f=w1322:u32)
            n227 = Select(t=w1324, s=w1320, f=w1323) -> (s? t:f=w1321:u32)
          }
          frame #2 {
            n228 = case shown="False" w1327 {
              frame #0 {
                w1330 = u32 0 ("APD 1 Counts 0")
                n229 = local write "APD 1 Counts 0"(w1330) -> ()
                n230 = local write "APD 2 Counts 0"(w1330) -> ()
              }
              frame #1 {
                w1331 = u32 0 ("APD 1 Counts 1")
                n231 = local write "APD 1 Counts 1"(w1331) -> ()
                n232 = local write "APD 2 Counts 1"(w1331) -> ()
              }
            }
          }
        }
      }
      frame #2 {
        n233 = feedback #17(w1365) -> (w1364:u32)
        n234 = Subtract(x=w1365, y=w1364) -> (x-y=w1363:u32)
        n235 = Subtract(x=w1363, y=w1362) -> (x-y=w1356:u32)
        n236 = case shown="True" "APD to FIFO" {
          tunnel: w1333 -> [_ w1392]
          tunnel: w1332 -> [_ w1390]
          frame #0 {
          }
          frame #1 {
            n237 = flat-sequence {
              tunnel: 0 ("Timeout") -> [w1394]
              tunnel: w1392 -> [w1395]
              tunnel: [w1394] -> w1391
              tunnel: w1391 -> [w1422]
              tunnel: w1390 -> [w1421]
              frame #0 {
                n238 = xnode ("FIFO Write")("Element"=w1395, "Timeout"=w1394) -> ()  [unwired: 1 in, 2 out]
              }
              frame #1 {
                n239 = xnode ("FIFO Write")("Element"=w1421, "Timeout"=w1422) -> ()  [unwired: 1 in, 2 out]
              }
            }
          }
        }
        n240 = Subtract(x="APD Acq Rate Count", y=w1356) -> (x-y=w1341:u32)
        n241 = Greater?(x=w1356, y=u32 0) -> (0:w1358:bool)
        "APD Acq Late?" <- w1358
        n242 = feedback #18(u32 0) -> (w1360:u32)
        n243 = Increment(x=w1360) -> (x+1=w1359:u32)
        n244 = Select(t=w1359, s=w1358, f=w1360) -> (s? t:f=w1357:u32)
        "APD Acq Late Counter" <- w1357
        n245 = Boolean To (0,1)(Boolean="+ phase (APD Acq)") -> (0, 1=w1337:i16)
        n246 = Multiply(x=w1337, y="Phase Count Adjustment (APD Acq)") -> (x*y=w1334:i16)
        n247 = Add(x=w1341, y=w1334) -> (x+y=w1340:u32)
        n248 = feedback #19(i16 0) -> (w1339:i16)
        n249 = Subtract(x=w1339, y=w1334) -> (x-y=w1336:i16)
        "APD Acq Relative Phase" <- w1336
        n250 = To Word Integer(number=w1333) -> (16bit integer=w1349:i16)
        n251 = To Word Integer(number=w1332) -> (16bit integer=w1350:i16)
        n252 = Multiply(x="APD 1 AO scale factor", y=w1349) -> (x*y=w1348:i16)
        n253 = Multiply(x="APD 2 AO scale factor", y=w1350) -> (x*y=w1347:i16)
        n254 = Add(x="APD 1 AO offset", y=w1348) -> (x+y=w1346:i16)
        n255 = Add(x=w1347, y="APD 2 AO offset") -> (x+y=w1344:i16)
        n256 = xnode "FPGA I/O Node"("Connector0/AO6"=w1346, "Connector0/AO7"=w1344) -> ()  [unwired: 2 in, 2 out]
      }
    }
  }
  n257 = while "MCL stage control" {
    shift-right: [w1463] -> _
    shift-left: w1 -> [w1466]
    shift-right: [w1456] -> _
    shift-left: w5 -> [w1453]
    shift-right: [w1455] -> _
    shift-left: w4 -> [w1451]
    i -> [w1450]
    stop <- FALSE stop-if-true
    n258 = flat-sequence {
      tunnel: w1466 -> [w1470]
      tunnel: [w1471] -> w1462
      tunnel: [w1470] -> w1460
      tunnel: [w1469] -> w1454
      tunnel: w1453 -> [w1469]
      tunnel: [w1468] -> w1452
      tunnel: w1451 -> [w1468]
      tunnel: w1462 -> [w1475]
      tunnel: [w1475] -> w1461
      tunnel: w1460 -> [w1474]
      tunnel: [w1474] -> w1459
      tunnel: w1454 -> [w1473]
      tunnel: w1452 -> [w1472]
      tunnel: [w1473] -> w1449
      tunnel: [w1472] -> w1448
      tunnel: w1461 -> [w1509]
      tunnel: w1459 -> [w1508]
      tunnel: [w1509] -> w1465
      tunnel: [w1508] -> w1464
      tunnel: [w1507] -> w1458
      tunnel: [w1506] -> w1457
      tunnel: w1449 -> [w1501]
      tunnel: w1448 -> [w1500]
      tunnel: [w1573] -> w1463
      tunnel: w1465 -> [w1587]
      tunnel: w1464 -> [w1584]
      tunnel: w1458 -> [w1576]
      tunnel: w1457 -> [w1575]
      tunnel: [w1576] -> w1456
      tunnel: [w1575] -> w1455
      frame #0 {
        n259 = call "Loop Timer5"("Count(Ticks)"=w1470) -> ("Tick Count(Ticks)"=w1471:u32)
      }
      frame #1 {
        n260 = xnode "FPGA I/O Node"("Connector0/AO1"=w1473, "Connector0/AO2"=w1472) -> ()  [unwired: 2 in, 2 out]
      }
      frame #2 {
        n261 = local read "Scanning MCL"() -> (w1521:bool)
        n262 = Or(x=w1521, y="Start scan (MCL)") -> (x .or. y?=w1516:bool)
        n263 = Not(x="Abort scan (MCL)") -> (.not. x?=w1514:bool)
        n264 = And(x=w1514, y=w1516) -> (x .and. y?=w1513:bool)
        n265 = case "Raster scan" shown="True" w1513 {
          tunnel: [w1522 w1565] -> w1518
          tunnel: "Start scan (MCL)" -> [_ w1550]
          tunnel: [w1522 w1526] -> w1502
          frame #0 {
            w1522 = i16 0
            n266 = local write "Scanning MCL"(FALSE ("scanning")) -> ()
          }
          frame #1 {
            w1536 = i16 0
            w1535 = u64 0
            # "scan incr."
            # "freq. incr. mult."
            # "count steps"
            # "count number of cycles"
            n267 = feedback #20(w1535) -> (w1562:u64)
            n268 = Select(t=w1535, s=w1550, f=w1562) -> (s? t:f=w1564:u64)
            n269 = Increment(x=w1564) -> (x+1=w1561:u64)
            n270 = Greater?(x="Cycles per step (MCL)", y=w1561) -> (0:w1545:bool)
            n271 = Select(t=w1561, s=w1545, f=w1535) -> (s? t:f=w1560:u64)
            n272 = feedback #21(w1535) -> (w1559:u64)
            n273 = Select(t=w1535, s=w1550, f=w1559) -> (s? t:f=w1554:u64)
            n274 = Increment(x=w1554) -> (x+1=w1558:u64)
            n275 = Add(x="Scan steps (MCL)", y="Scan steps (MCL)") -> (x+y=w1557:u64)
            n276 = Select(t=w1554, s=w1545, f=w1558) -> (s? t:f=w1540:u64)
            n277 = Greater?(x=w1557, y=w1540) -> (0:w1539:bool)
            n278 = Select(t=w1540, s=w1539, f=w1535) -> (s? t:f=w1555:u64)
            n279 = Equal?(x="Scan steps (MCL)", y=w1540) -> (x = y?=w1544:bool)
            n280 = Greater?(x="Scan steps (MCL)", y=w1554) -> (0:w1553:bool)
            n281 = feedback #22(w1536) -> (w1556:i16)
            n282 = Select(t=w1536, s=w1550, f=w1556) -> (s? t:f=w1542:i16)
            n283 = Increment(x=w1542) -> (x+1=w1552:i16)
            n284 = Decrement(x=w1542) -> (x-1=w1551:i16)
            n285 = Select(t=w1552, s=w1553, f=w1551) -> (s? t:f=w1543:i16)
            n286 = Select(t=w1542, s=w1544, f=w1543) -> (s? t:f=w1541:i16)
            n287 = Select(t=w1542, s=w1545, f=w1541) -> (s? t:f=w1537:i16)
            n288 = Select(t=w1537, s=w1539, f=w1536) -> (s? t:f=w1538:i16)
            n289 = feedback #23(w1535) -> (w1549:u64)
            n290 = Select(t=w1535, s=w1550, f=w1549) -> (s? t:f=w1524:u64)
            n291 = Increment(x=w1524) -> (x+1=w1546:u64)
            n292 = Select(t=w1524, s=w1539, f=w1546) -> (s? t:f=w1525:u64)
            n293 = Greater?(x="Number of scans (MCL)", y=w1525) -> (0:w1532:bool)
            n294 = Multiply(x="Scan freq.  increment (MCL)", y=w1542) -> (x*y=w1565:i16)
            n295 = Select(t=TRUE, s="Cont. Scan (MCL)", f=w1532) -> (s? t:f=w1531:bool)
            "Scanning MCL" <- w1531
            n296 = Select(t=w1525, s=w1531, f=w1535) -> (s? t:f=w1547:u64)
            n297 = Increment(x=w1525) -> (x+1=→"Scan I (MCL)":u64)
            n298 = To Word Integer(number=w1524) -> (16bit integer=w1527:i16)
            n299 = Multiply(x=w1527, y="Scan freq.  increment (MCL)") -> (x*y=w1526:i16)
          }
        }
        n300 = Select(t=w1502, s="1D or 2D Scan?", f=i16 0) -> (s? t:f=w1503:i16)
        n301 = Select(t=w1503, s="MCL Scan Axis", f=w1518) -> (s? t:f=w1517:i16)
        n302 = Select(t=w1518, s="MCL Scan Axis", f=w1503) -> (s? t:f=w1519:i16)
        n303 = Add(x=w1517, y="AO2") -> (x+y=w1506:i16)
        n304 = Add(x="AO1", y=w1519) -> (x+y=w1507:i16)
        "AO1 2" <- w1501
        "AO2 2" <- w1500
      }
      frame #3 {
        n305 = feedback #24(w1587) -> (w1586:u32)
        n306 = Boolean To (0,1)(Boolean="+ phase (MCL)") -> (0, 1=w1571:i16)
        n307 = Subtract(x=w1587, y=w1586) -> (x-y=w1585:u32)
        n308 = Multiply(x=w1571, y="Phase count adjustment (MCL)") -> (x*y=w1567:i16)
        n309 = Subtract(x=w1585, y=w1584) -> (x-y=w1582:u32)
        n310 = Subtract(x="MCL count", y=w1582) -> (x-y=w1569:u32)
        n311 = feedback #25(i16 0) -> (w1568:i16)
        n312 = Subtract(x=w1568, y=w1567) -> (x-y=w1566:i16)
        "MCL Relative Phase" <- w1566
        n313 = Greater?(x=w1582, y=u32 0) -> (0:w1581:bool)
        "MCL Late?" <- w1581
        n314 = Add(x=w1569, y=w1567) -> (x+y=w1573:u32)
        n315 = feedback #26(u32 0) -> (w1579:u32)
        n316 = Increment(x=w1579) -> (x+1=w1578:u32)
        n317 = Select(t=w1578, s=w1581, f=w1579) -> (s? t:f=w1580:u32)
        "MCL Late Counter" <- w1580
      }
    }
    "Numeric" <- w1450
  }
  n318 = while "APD Gating" {
    shift-right: [w1592] -> _
    shift-left: w1 -> [w1597]
    shift-right: [w1591] -> _
    shift-left: FALSE -> [w1589]
    stop <- FALSE stop-if-true
    n319 = flat-sequence {
      tunnel: w1597 -> [w1600]
      tunnel: [w1601] -> w1595
      tunnel: [w1600] -> w1593
      tunnel: [w1599] -> w1590
      tunnel: w1589 -> [w1599]
      tunnel: [w1604] -> w1596
      tunnel: w1595 -> [w1604]
      tunnel: [w1603] -> w1594
      tunnel: w1593 -> [w1603]
      tunnel: w1590 -> [w1602]
      tunnel: [w1714] -> w1592
      tunnel: w1596 -> [w1736]
      tunnel: w1594 -> [w1733]
      tunnel: [w1719] -> w1591
      frame #0 {
        n320 = call "Loop Timer7"("Count(Ticks)"=w1600) -> ("Tick Count(Ticks)"=w1601:u32)
      }
      frame #1 {
        # "Can switch 2 APDs\n(need 4 channels/APD)"
        n321 = xnode "FPGA I/O Node"("Connector0/DIO0"=w1602, "Connector0/DIO1"=w1602, "Connector0/DIO2"=w1602, "Connector0/DIO3"=w1602, "Connector0/DIO4"=w1602, "Connector0/DIO5"=w1602, "Connector0/DIO6"=w1602, "Connector0/DIO7"=w1602) -> ()  [unwired: 8 in, 8 out]
      }
      frame #2 {
        n322 = feedback #27(TRUE) -> (w1722:bool)
        n323 = feedback #28(w1736) -> (w1735:u32)
        n324 = Not(x=w1722) -> (.not. x?=w1718:bool)
        n325 = Subtract(x=w1736, y=w1735) -> (x-y=w1734:u32)
        n326 = Select(t="APD Gate ON Count", s=w1718, f="APD Gate OFF Count") -> (s? t:f=w1724:u32)
        n327 = Subtract(x=w1734, y=w1733) -> (x-y=w1725:u32)
        n328 = Subtract(x=w1724, y=w1725) -> (x-y=w1713:u32)
        n329 = Greater?(x=w1725, y=u32 0) -> (0:w1729:bool)
        "APD Gate Late?" <- w1729
        n330 = Boolean To (0,1)(Boolean="+ phase (APD Gate)") -> (0, 1=w1711:i16)
        n331 = Multiply(x=w1711, y="Phase count adjustment (APD Gate)") -> (x*y=w1709:i16)
        n332 = feedback #29(u32 0) -> (w1731:u32)
        n333 = Increment(x=w1731) -> (x+1=w1730:u32)
        n334 = Select(t=w1730, s=w1729, f=w1731) -> (s? t:f=w1728:u32)
        "APD Gate Late Counter" <- w1728
        n335 = Add(x=w1713, y=w1709) -> (x+y=w1714:u32)
        n336 = feedback #30(i16 0) -> (w1716:i16)
        n337 = Subtract(x=w1716, y=w1709) -> (x-y=w1715:i16)
        "APD Gate Relative Phase" <- w1715
        n338 = case shown="2" "APD Gate Operating Mode" {
          tunnel: [TRUE FALSE w1742] -> w1719
          tunnel: w1722 -> [_ _ w1739]
          frame #0 {
          }
          frame #1 {
          }
          frame #2 {
            n339 = Not(x=w1739) -> (.not. x?=w1741:bool)
            n340 = Select(t=w1741, s="Invert APD Gate", f=w1739) -> (s? t:f=w1742:bool)
          }
        }
      }
    }
  }
  n341 = while "Green excitation laser feedback measurement" {
    shift-right: [w1743] -> _
    shift-left: w1 -> [w1748]
    stop <- FALSE stop-if-true
    n342 = flat-sequence {
      tunnel: w1748 -> [w1750]
      tunnel: [w1751] -> w1746
      tunnel: [w1750] -> w1744
      tunnel: [w1758] -> w1747
      tunnel: w1746 -> [w1758]
      tunnel: [w1757] -> w1745
      tunnel: w1744 -> [w1757]
      tunnel: [w1834] -> w1743
      tunnel: w1747 -> [w1852]
      tunnel: w1745 -> [w1849]
      frame #0 {
        n343 = call "Loop Timer9"("Count(Ticks)"=w1750) -> ("Tick Count(Ticks)"=w1751:u32)
      }
      frame #1 {
        n344 = xnode "FPGA I/O Node"("Connector1/DIO35"=TRUE) -> ("Chassis2/Mod1/AI0"=w1756:i16, "Chassis2/Mod1/AI1"=w1755:i16, "Chassis2/Mod1/AI2"=w1752:i16)  [unwired: 4 in, 4 out]
        "Green FB Sum" <- w1752
        n345 = Bundle("Chassis2/Mod1/AI0"=w1756, "Chassis2/Mod1/AI1"=w1755, "Chassis2/Mod1/AI2"=w1752) -> (→"Green FB Signals":T12)  [unwired: 1 out]
      }
      frame #2 {
        n346 = feedback #31(w1852) -> (w1851:u32)
        n347 = Subtract(x=w1852, y=w1851) -> (x-y=w1850:u32)
        n348 = xnode "FPGA I/O Node"("Connector1/DIO35"=FALSE) -> ()  [unwired: 1 in, 1 out]
        n349 = Subtract(x=w1850, y=w1849) -> (x-y=w1843:u32)
        n350 = Subtract(x="Green FB Count", y=w1843) -> (x-y=w1838:u32)
        n351 = Greater?(x=w1843, y=u32 0) -> (0:w1845:bool)
        "Green FB Late?" <- w1845
        n352 = Boolean To (0,1)(Boolean="+ phase (Green FB)") -> (0, 1=w1836:i16)
        n353 = Multiply(x=w1836, y="Phase count adjustment (Green FB)") -> (x*y=w1831:i16)
        n354 = feedback #32(u32 0) -> (w1847:u32)
        n355 = Increment(x=w1847) -> (x+1=w1846:u32)
        n356 = Select(t=w1846, s=w1845, f=w1847) -> (s? t:f=w1844:u32)
        "Green Late Counter" <- w1844
        n357 = Add(x=w1838, y=w1831) -> (x+y=w1834:u32)
        n358 = feedback #33(i16 0) -> (w1833:i16)
        n359 = Subtract(x=w1833, y=w1831) -> (x-y=w1832:i16)
        "Green FB Relative Phase" <- w1832
      }
    }
  }
  n360 = while "Green fluorescent laser interlacing (DO to IA 532 nm AOM ME amp)." {
    shift-right: [w1868] -> _
    shift-left: w1 -> [w1873]
    shift-right: [w1867] -> _
    shift-left: FALSE -> [w1865]
    stop <- FALSE stop-if-true
    n361 = flat-sequence {
      tunnel: w1873 -> [w1876]
      tunnel: [w1877] -> w1871
      tunnel: [w1876] -> w1869
      tunnel: [w1875] -> w1866
      tunnel: w1865 -> [w1875]
      tunnel: [w1880] -> w1872
      tunnel: w1871 -> [w1880]
      tunnel: [w1879] -> w1870
      tunnel: w1869 -> [w1879]
      tunnel: w1866 -> [w1878]
      tunnel: [w1920] -> w1868
      tunnel: w1872 -> [w1947]
      tunnel: w1870 -> [w1944]
      tunnel: [w1930] -> w1867
      frame #0 {
        n362 = call "Loop Timer4"("Count(Ticks)"=w1876) -> ("Tick Count(Ticks)"=w1877:u32)
      }
      frame #1 {
        n363 = xnode "FPGA I/O Node"("Connector1/DIO37"=w1878, "Connector1/DIO38"=w1878, "Connector1/DIO39"=w1878) -> ()  [unwired: 3 in, 3 out]
      }
      frame #2 {
        n364 = feedback #34(w1947) -> (w1946:u32)
        n365 = Subtract(x=w1947, y=w1946) -> (x-y=w1945:u32)
        n366 = Subtract(x=w1945, y=w1944) -> (x-y=w1936:u32)
        n367 = Greater?(x=w1936, y=u32 0) -> (0:w1940:bool)
        "GI Late?" <- w1940
        n368 = Boolean To (0,1)(Boolean="+ phase (GI)") -> (0, 1=w1925:i16)
        n369 = Multiply(x=w1925, y="Phase count adjustment (GI)") -> (x*y=w1922:i16)
        n370 = feedback #35(u32 0) -> (w1942:u32)
        n371 = Increment(x=w1942) -> (x+1=w1941:u32)
        n372 = Select(t=w1941, s=w1940, f=w1942) -> (s? t:f=w1939:u32)
        "GI Late Counter" <- w1939
        n373 = feedback #36(i16 0) -> (w1923:i16)
        n374 = Subtract(x=w1923, y=w1922) -> (x-y=w1921:i16)
        "GI Relative phase" <- w1921
        n375 = feedback #37(TRUE) -> (w1933:bool)
        n376 = case shown="2" "Operating Mode" {
          tunnel: [TRUE FALSE w1953] -> w1930
          tunnel: w1933 -> [_ _ w1950]
          frame #0 {
          }
          frame #1 {
          }
          frame #2 {
            n377 = Not(x=w1950) -> (.not. x?=w1952:bool)
            n378 = Select(t=w1952, s="Invert GI", f=w1950) -> (s? t:f=w1953:bool)
          }
        }
        n379 = Not(x=w1933) -> (.not. x?=w1929:bool)
        n380 = Select(t="Green interlace ON count", s=w1929, f="Green interlace OFF count") -> (s? t:f=w1935:u32)
        n381 = Subtract(x=w1935, y=w1936) -> (x-y=w1926:u32)
        n382 = Add(x=w1926, y=w1922) -> (x+y=w1920:u32)
      }
    }
  }
  n383 = while "Green fluorescent laser interlacing (Current to IA 532 nm AOM ME amp)." {
    shift-right: [w1959] -> _
    shift-left: w1 -> [w1962]
    shift-right: [w1956] -> _
    shift-left: w1 -> [w1954]
    stop <- FALSE stop-if-true
    n384 = flat-sequence {
      tunnel: w1962 -> [w1965]
      tunnel: [w1966] -> w1961
      tunnel: [w1965] -> w1960
      tunnel: [w1964] -> w1955
      tunnel: w1954 -> [w1964]
      tunnel: [w1969] -> w1958
      tunnel: w1961 -> [w1969]
      tunnel: [w1968] -> w1957
      tunnel: w1960 -> [w1968]
      tunnel: w1955 -> [w1967]
      tunnel: [w1982] -> w1959
      tunnel: [w2000] -> w1956
      tunnel: w1958 -> [w2019]
      tunnel: w1957 -> [w2016]
      frame #0 {
        n385 = call "Loop Timer10"("Count(Ticks)"=w1965) -> ("Tick Count(Ticks)"=w1966:u32)
      }
      frame #1 {
        n386 = xnode "FPGA I/O Node"("Chassis2/Mod4/AO0"=w1967) -> ()  [unwired: 1 in, 1 out]
      }
      frame #2 {
        n387 = Subtract(x="Green interlace OFF count 2", y="Green int current ON count adj") -> (x-y=w1992:u32)
        n388 = feedback #38(w2019) -> (w2018:u32)
        n389 = Add(x="Green int current ON count adj", y="Green interlace ON count 2") -> (x+y=w1993:u32)
        n390 = Subtract(x=w2019, y=w2018) -> (x-y=w2017:u32)
        n391 = Subtract(x=w2017, y=w2016) -> (x-y=w2008:u32)
        n392 = Greater?(x=w2008, y=u32 0) -> (0:w2012:bool)
        "GI Late? 2" <- w2012
        n393 = Boolean To (0,1)(Boolean="+ phase (GI) 2") -> (0, 1=w1988:i16)
        n394 = Multiply(x=w1988, y="Phase count adjustment (GI) 2") -> (x*y=w1984:i16)
        n395 = feedback #39(u32 0) -> (w2014:u32)
        n396 = Increment(x=w2014) -> (x+1=w2013:u32)
        n397 = Select(t=w2013, s=w2012, f=w2014) -> (s? t:f=w2011:u32)
        "GI Late Counter 2" <- w2011
        n398 = feedback #40(i16 0) -> (w1985:i16)
        n399 = Subtract(x=w1985, y=w1984) -> (x-y=w1983:i16)
        "GI Relative phase 2" <- w1983
        n400 = feedback #41(TRUE) -> (w2005:bool)
        n401 = case shown="2" "Operating Mode 2" {
          tunnel: [TRUE FALSE w2036] -> w1994
          tunnel: w2005 -> [_ _ w2033]
          frame #0 {
          }
          frame #1 {
          }
          frame #2 {
            n402 = Not(x=w2033) -> (.not. x?=w2035:bool)
            n403 = Select(t=w2035, s="Invert GI 2", f=w2033) -> (s? t:f=w2036:bool)
          }
        }
        n404 = And(x=w1994, y="Green FB On/Off") -> (x .and. y?=w1995:bool)
        n405 = case shown="True" w1995 {
          tunnel: "Current Out" -> [w2020 _]
          tunnel: [w2020 w2025] -> w1999
          frame #0 {
          }
          frame #1 {
            n406 = local read "Green FB Sum"() -> (w2021:i16)
            n407 = call "Slower PID.vi"("process variable"=w2021, "reset?"="Green FB Reset", "setpoint"="Green FB Setpoint", "PID gains (x 2^8)"="Green FB Gains", "output range"=cluster{"output high":i16, "output low":i16} {"output high"=32767, "output low"=-32768} ("Green FB output range")) -> ("output"=w2029:i16)  [unwired: 10 out]
            n408 = To Long Integer(number=w2029) -> (32bit integer=w2022:i32)
            n409 = Add(x=w2022, y=32768) -> (x+y=w2024:i32)
            n410 = To Unsigned Word Integer(number=w2024) -> (unsigned 16bit integer=w2025:u16)
          }
        }
        n411 = Not(x=w2005) -> (.not. x?=w2002:bool)
        n412 = Select(t=w1993, s=w2002, f=w1992) -> (s? t:f=w2007:u32)
        n413 = Subtract(x=w2007, y=w2008) -> (x-y=w1986:u32)
        n414 = Add(x=w1986, y=w1984) -> (x+y=w1982:u32)
        n415 = Boolean To (0,1)(Boolean=w1994) -> (0, 1=w2001:i16)
        n416 = To Unsigned Word Integer(number=w2001) -> (unsigned 16bit integer=w1998:u16)
        n417 = Multiply(x=w1998, y=w1999) -> (x*y=w2000:u16)
      }
    }
  }
  n418 = while "RF box board direct communication loop" {
    tunnel: w1 -> [_]
    stop <- FALSE stop-if-true
    n419 = case "Whether to use direct communication method (only use one method at a time)" shown="True" "Direct RF Box \nCommunication" {
      frame #0 {
      }
      frame #1 {
        n420 = case shown="True" "Update Data" {
          frame #0 {
          }
          frame #1 {
            n421 = flat-sequence {
              frame #0 {
                n422 = First Call?() -> (First Call?: T/F=w2040:bool)
                n423 = case shown="True" w2040 {
                  frame #0 {
                  }
                  frame #1 {
                    # "If first time data updated, be sure to set WR high\nbefore setting data and address bits."
                    n424 = flat-sequence {
                      frame #0 {
                        n425 = xnode "FPGA I/O Node"("Connector1/DIO15"=TRUE) -> ()  [unwired: 1 in, 1 out]
                      }
                      frame #1 {
                        n426 = call "Wait"("Count(Ticks)"=u8 40 ("DO Delay 3 (Ticks)")) -> ()  [unwired: 1 out]
                      }
                    }
                  }
                }
              }
              frame #1 {
                n427 = Number To Boolean Array(number="Address") -> (Boolean array=w2102:bool[])
                n428 = Number To Boolean Array(number="Data BD 1") -> (Boolean array=w2103:bool[])
                n429 = Number To Boolean Array(number="Data BD 2") -> (Boolean array=w2072:bool[])
                n430 = Index Array(array=w2103, index=7) -> (element=w2087:bool)
                n431 = Index Array(array=w2103, index=6) -> (element=w2086:bool)
                n432 = Index Array(array=w2103, index=5) -> (element=w2085:bool)
                n433 = Index Array(array=w2103, index=4) -> (element=w2084:bool)
                n434 = Index Array(array=w2103, index=3) -> (element=w2083:bool)
                n435 = Index Array(array=w2103, index=2) -> (element=w2082:bool)
                n436 = Index Array(array=w2103, index=1) -> (element=w2081:bool)
                n437 = Index Array(array=w2103, index=0) -> (element=w2080:bool)
                n438 = Index Array(array=w2102, index=5) -> (element=w2079:bool)
                n439 = Index Array(array=w2102, index=4) -> (element=w2078:bool)
                n440 = Index Array(array=w2102, index=3) -> (element=w2077:bool)
                n441 = Index Array(array=w2102, index=2) -> (element=w2076:bool)
                n442 = Index Array(array=w2102, index=1) -> (element=w2075:bool)
                n443 = Index Array(array=w2102, index=0) -> (element=w2074:bool)
                n444 = Index Array(array=w2072, index=7) -> (element=w2063:bool)
                n445 = Index Array(array=w2072, index=6) -> (element=w2062:bool)
                n446 = Index Array(array=w2072, index=5) -> (element=w2061:bool)
                n447 = Index Array(array=w2072, index=4) -> (element=w2060:bool)
                n448 = Index Array(array=w2072, index=3) -> (element=w2059:bool)
                n449 = Index Array(array=w2072, index=2) -> (element=w2058:bool)
                n450 = Index Array(array=w2072, index=1) -> (element=w2057:bool)
                n451 = Index Array(array=w2072, index=0) -> (element=w2056:bool)
                n452 = xnode "FPGA I/O Node"("Connector1/DIO0"=w2087, "Connector1/DIO1"=w2086, "Connector1/DIO2"=w2085, "Connector1/DIO3"=w2084, "Connector1/DIO4"=w2083, "Connector1/DIO5"=w2082, "Connector1/DIO6"=w2081, "Connector1/DIO7"=w2080, "Connector1/DIO8"=w2079, "Connector1/DIO9"=w2078, "Connector1/DIO10"=w2077, "Connector1/DIO11"=w2076, "Connector1/DIO12"=w2075, "Connector1/DIO13"=w2074, "Connector1/DIO20"=w2063, "Connector1/DIO21"=w2062, "Connector1/DIO22"=w2061, "Connector1/DIO23"=w2060, "Connector1/DIO24"=w2059, "Connector1/DIO25"=w2058, "Connector1/DIO26"=w2057, "Connector1/DIO27"=w2056) -> ()  [unwired: 22 in, 22 out]
              }
              frame #2 {
                # "wait and then apply write signal"
                n453 = call "Wait2"("Count(Ticks)"=u8 40 ("DO Delay 1 (Ticks)")) -> ()  [unwired: 1 out]
              }
              frame #3 {
                # "sending bit low writes data to board buffer"
                n454 = xnode "FPGA I/O Node"("Connector1/DIO15"=FALSE) -> ()  [unwired: 1 in, 1 out]
              }
              frame #4 {
                # "wait then return write signal"
                n455 = call "Wait3"("Count(Ticks)"=u8 40 ("DO Delay 2 (Ticks)")) -> ()  [unwired: 1 out]
              }
              frame #5 {
                # "sending bit high makes ready to\nwrite more data"
                n456 = xnode "FPGA I/O Node"("Connector1/DIO15"=TRUE) -> ()  [unwired: 1 in, 1 out]
              }
            }
          }
        }
      }
    }
  }
  n457 = node-c288(w2) -> ()
